vi "destroy notifiers.vi"(11 "Template in":refnum<class "Template.lvclass">) -> (3 "Template out":refnum<class "Template.lvclass">)   [LabVIEW 2020, in "Template.lvlib" / "Template.lvclass"]
uses:
  Template.lvclass
  Template.lvclass/Template.ctl
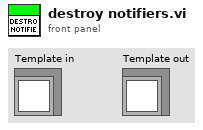
[diagram p1: front panel]
types:
  T1 = typedef "Template.lvlib/Template.lvclass/base actor notifiers.ctl" = cluster{"Stop Actor":refnum<notifier>}
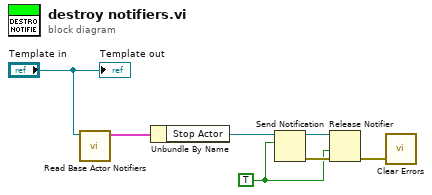
[diagram p0: block diagram]
diagram:
  w1 = TRUE ("notification")
  n1 = call "Read Base Actor Notifiers.vi"("Template in"="Template in") -> ("Base Actor Notifiers"=w6:T1)  [unwired: 10 in]
  n2 = Unbundle By Name(w6) -> ("Stop Actor"=w5:refnum<notifier>)
  n3 = Send Notification(notification=w1, notifier=w5) -> (notifier out=w3:refnum<notifier>, error out=w2:errorcluster)  [unwired: 1 in]
  n4 = Release Notifier(notifier=w3, force destroy? (F)=w1, error in (no error)=w2) -> (error out=w4:errorcluster)  [unwired: 2 out]
  n5 = call <vilib>:"Clear Errors.vi"("error in (no error)"=w4) -> ()  [unwired: 5 in, 2 out]
  "Template out" <- "Template in"
